vi "Heat2D_X Neumann Type.vi"(0 "BC Value(n+1)":dbl[](array[numeric]), 1 "Left?":bool=TRUE, 5 "BC Value(n)":dbl[](array[numeric]), 7 "Coefficients":T1, 9 "F(n+1)+F(n)":dbl[](array[numeric]), 11 "Extended U(n)":dbl[][](array[numeric])) -> (4 "RHS":dbl[](array[numeric]))   [LabVIEW 2017, in "NI_PDE.lvlib"]
uses:
  <vilib>/gmath/NI_PDE.lvlib
  <vilib>/Analysis/2dsp.llb/1D Convolution (DBL).vi
  <vilib>/Analysis/NI_AALPro.lvlib
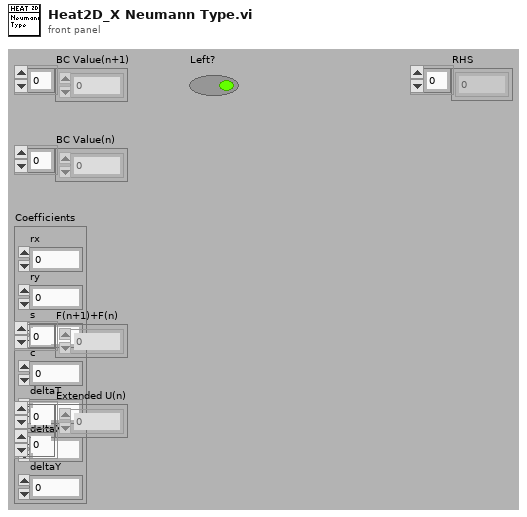
[diagram p1: front panel]
types:
  T1 = cluster{"rx":dbl, "ry":dbl, "s":dbl, "c":dbl, "deltaT":dbl, "deltaX":dbl, "deltaY":dbl}
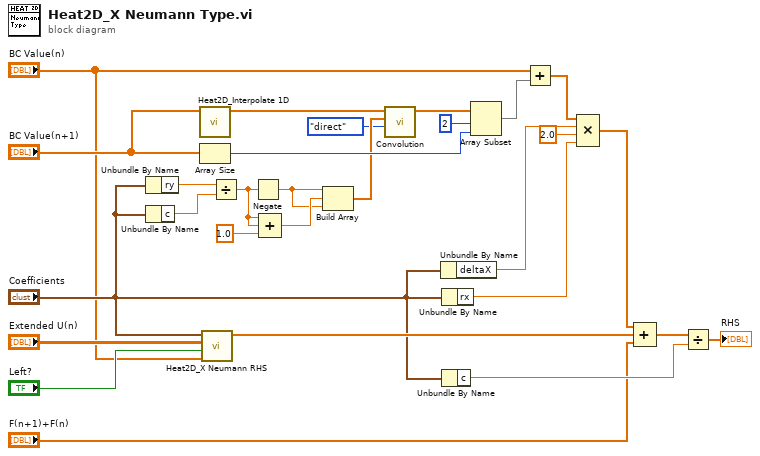
[diagram p0: block diagram]
diagram:
  n1 = Unbundle By Name("Coefficients") -> ("ry"=w14:dbl)
  n2 = Unbundle By Name("Coefficients") -> ("c"=w12:dbl)
  n3 = call <vilib>:"Heat2D_Interpolate 1D.vi"("X"="BC Value(n+1)") -> ("Interp(X)"=w20:dbl[])  [unwired: 1 in, 9 out]
  n4 = Array Size(array="BC Value(n+1)") -> (size(s)=w18:i32)
  n5 = call <vilib>:"Heat2D_X Neumann RHS.vi"("BC Value(n)"="BC Value(n)", "Left?"="Left?", "Extended U(n)"="Extended U(n)", "Coefficients"="Coefficients") -> ("RHS vector"=w8:dbl[])  [unwired: 7 out]
  n6 = Divide(x=w14, y=w12) -> (x/y=w28:dbl)
  n7 = Negate(x=w28) -> (-x=w25:dbl)
  n8 = Compound Arithmetic op=ADD(w28, w28, 1.0 ("value")) -> (w26:dbl)
  n9 = Build Array(w25, w26, w25) -> (w17:dbl[])
  n10 = call-poly <vilib>:"Convolution.vi"("algorithm"=enum32{"direct", "frequency domain"}."direct", "Y"=w17, "X"=w20) -> ("X * Y"=w22:dbl[])  [unwired: 8 out]
  n11 = Unbundle By Name("Coefficients") -> ("deltaX"=w23:dbl)
  n12 = Unbundle By Name("Coefficients") -> ("rx"=w9:dbl)
  n13 = Unbundle By Name("Coefficients") -> ("c"=w6:dbl)
  n14 = Array Subset(array=w22, index=2, length=w18) -> (w5:dbl[])
  n15 = Add(x="BC Value(n)", y=w5) -> (x+y=w4:dbl[])
  n16 = Compound Arithmetic op=MULTIPLY(w4, w23, 2.0 ("value"), w9) -> (w24:dbl[])
  n17 = Compound Arithmetic op=ADD(w24, w8, "F(n+1)+F(n)") -> (w13:dbl[])
  n18 = Divide(x=w13, y=w6) -> (x/y=→"RHS":dbl[])
